vi "PCC Main.vi"(10 "Data Type DVRs":T1, 11 "Config Folder":path) -> ()   [LabVIEW 2018]
uses:
  Controls/State Transition Loop Selector.ctl
  Controls/DDS State.ctl
  <vilib>/ORNL/CSEISMIC DDS/CSEISMIC DDS Base/Data Types/Controls/DeviceID.ctl
  Controls/Data Type DVRs.ctl
  <vilib>/ORNL/CSEISMIC DDS/CSEISMIC DDS Base/Data Types/PCC_Transition.ctl
  <vilib>/ORNL/CSEISMIC DDS/CSEISMIC DDS Base/Data Types/Controls/Timestamp.ctl
  <vilib>/ORNL/CSEISMIC DDS/CSEISMIC DDS Base/Data Types/DER_setGenerationMode.ctl
  <vilib>/ORNL/CSEISMIC DDS/CSEISMIC DDS Base/Data Types/Controls/Generation Mode.ctl
  <vilib>/ORNL/CSEISMIC DDS/CSEISMIC DDS Base/Data Types/IED_Status.ctl
  <vilib>/ORNL/CSEISMIC DDS/CSEISMIC DDS Base/Data Types/DER_VF.ctl
  <vilib>/ORNL/CSEISMIC DDS/CSEISMIC DDS Base/Data Types/SmartRelay_Measurement.ctl
  5fae7271-6999-4ee3-adec-77b7e82a9117.vi
  0c60829f-05e1-488a-9307-f5885f688830.vi
  d2d44614-09ee-478f-a8ad-1eeb43ba122a.vi
  90de438a-d49d-4198-a24f-55d882466989.vi
  1e39ed10-ef24-4d6c-8bee-b3eb3189697a.vi
  ae37c20a-06b2-40c0-9558-581a6213f2f7.vi
  c6f44c25-c2e0-4f56-a5f0-2cf136f07edc.vi
  86f4f49e-388a-4250-a9a8-ce7cd87dfdd2.vi
  05904c7c-c053-4fcf-9d3f-90a477ff682e.vi
  6fac8efd-f310-42bf-8d4e-08964d51a696.vi
  85c23227-e024-4d6f-8611-baa9cc794223.vi
  278e74c7-9ea8-40bf-a49e-ca8128e71b27.vi
  9b8a6be7-b97e-4c02-9044-44fe14d12b33.vi
  Global Variables/Stop (Global).vi
  Global Variables/DDS States (Global).vi
  Global Variables/Manual Control (Global).vi
  Global Variables/Measurements (Global).vi
  <vilib>/ORNL/CSEISMIC DDS/CSEISMIC DDS Base/CSEISMIC DDS.lvclass
  <vilib>/ptbypt/NI_PtbyPt.lvlib
  <vilib>/Analysis/NI_AALBase.lvlib
panel:
  out "Switch Closed?":bool=TRUE
  out "VF DeviceID":T2
  out "MicrogridID":u8
  out "Error in DDS Loop":bool
  out "DDS Error out":errorcluster
  out "DDS State":T3
  out "DDS loop time":u32=100
  out "Error in State Transition Loop":bool
  out "DDS state m/c loop time":u32=100
  out "Trans State":T4
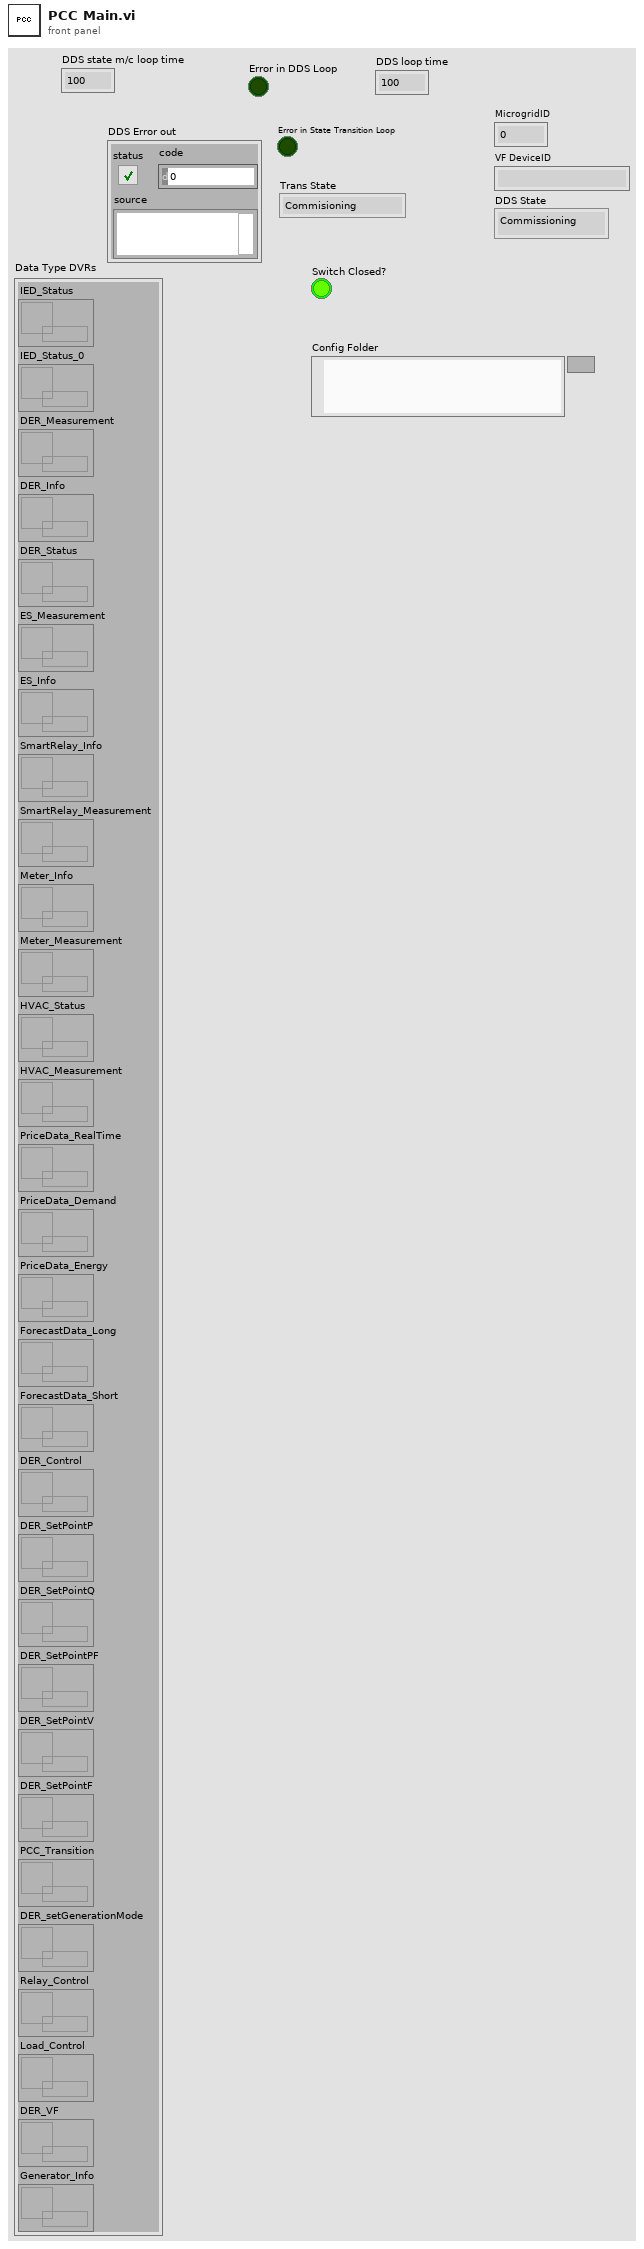
[diagram p1: front panel]
types:
  T1 = typedef "Data Type DVRs.ctl" = cluster{"IED_Status":refnum<data-value>, "IED_Status_0":refnum<data-value>, "DER_Measurement":refnum<data-value>, "DER_Info":refnum<data-value>, "DER_Status":refnum<data-value>, "ES_Measurement":refnum<data-value>, "ES_Info":refnum<data-value>, "SmartRelay_Info":refnum<data-value>, "SmartRelay_Measurement":refnum<data-value>, "Meter_Info":refnum<data-value>, "Meter_Measurement":refnum<data-value>, "HVAC_Status":refnum<data-value>, "HVAC_Measurement":refnum<data-value>, "PriceData_RealTime":refnum<data-value>, "PriceData_Demand":refnum<data-value>, "PriceData_Energy":refnum<data-value>, "ForecastData_Long":refnum<data-value>, "ForecastData_Short":refnum<data-value>, "DER_Control":refnum<data-value>, "DER_SetPointP":refnum<data-value>, "DER_SetPointQ":refnum<data-value>, "DER_SetPointPF":refnum<data-value>, "DER_SetPointV":refnum<data-value>, "DER_SetPointF":refnum<data-value>, "PCC_Transition":refnum<data-value>, "DER_setGenerationMode":refnum<data-value>, "Relay_Control":refnum<data-value>, "Load_Control":refnum<data-value>, "DER_VF":refnum<data-value>, "Generator_Info":refnum<data-value>}
  T2 = typedef "CSEISMIC DDS.lvlib/CSEISMIC DDS.lvclass/DeviceID.ctl" = string
  T3 = typedef "DDS State.ctl" = enum16{"Commissioning", "CheckID", "InitDDS", "ReadDDS", "WriteDDS", "CheckClose", "Close", "Shutdown"}
  T4 = typedef "State Transition Loop Selector.ctl" = enum16{"Commisioning", "Start", "Open", "Closed", "Resynch", "Island", "Close References", "Shutdown"}
  T5 = typedef "Smart Relay Config Settings.ctl" = cluster{"ResynchTimeout":dbl, "IslandTimeout":dbl}
  T6 = typedef "CSEISMIC DDS.lvlib/CSEISMIC DDS.lvclass/SmartRelay_Info.ctl" = cluster{"DeviceID":T2, "LineConfig":u8[], "NominalVoltage(V)":dbl}
  T7 = typedef "CSEISMIC DDS.lvlib/CSEISMIC DDS.lvclass/Timestamp.ctl" = cluster{"Seconds":u64, "Remainder":u64}
  T8 = typedef "CSEISMIC DDS.lvlib/CSEISMIC DDS.lvclass/IED_Status.ctl" = cluster{"DeviceID":T2, "Timestamp":T7, "MicrogridID":u8, "Active":bool, "Inactive":bool, "Error":i32, "Fault":bool, "ErrorString":string}
  T9 = typedef "CSEISMIC DDS.lvlib/CSEISMIC DDS.lvclass/DER_VF.ctl" = cluster{"DeviceID":T2}
  T10 = typedef "CSEISMIC DDS.lvlib/CSEISMIC DDS.lvclass/SmartRelay_Measurement.ctl" = cluster{"DeviceID":T2, "PrimaryVoltage":dbl[], "SecondaryVoltage":dbl[], "Current":dbl[], "RealPower":dbl[], "ReactivePower":dbl[], "LineConfig":u8[], "Frequency":dbl}
  T11 = typedef "CSEISMIC DDS.lvlib/CSEISMIC DDS.lvclass/PCC_Transition.ctl" = cluster{"DeviceID":T2, "Island":bool, "Resynchronize":bool}
  T12 = typedef "CSEISMIC DDS.lvlib/CSEISMIC DDS.lvclass/Generation Mode.ctl" = enum32{"Invalid", "PQ", "Droop", "PV", "PF", "VF"}
  T13 = typedef "CSEISMIC DDS.lvlib/CSEISMIC DDS.lvclass/DER_setGenerationMode.ctl" = cluster{"DeviceID":T2, "Mode":T12}
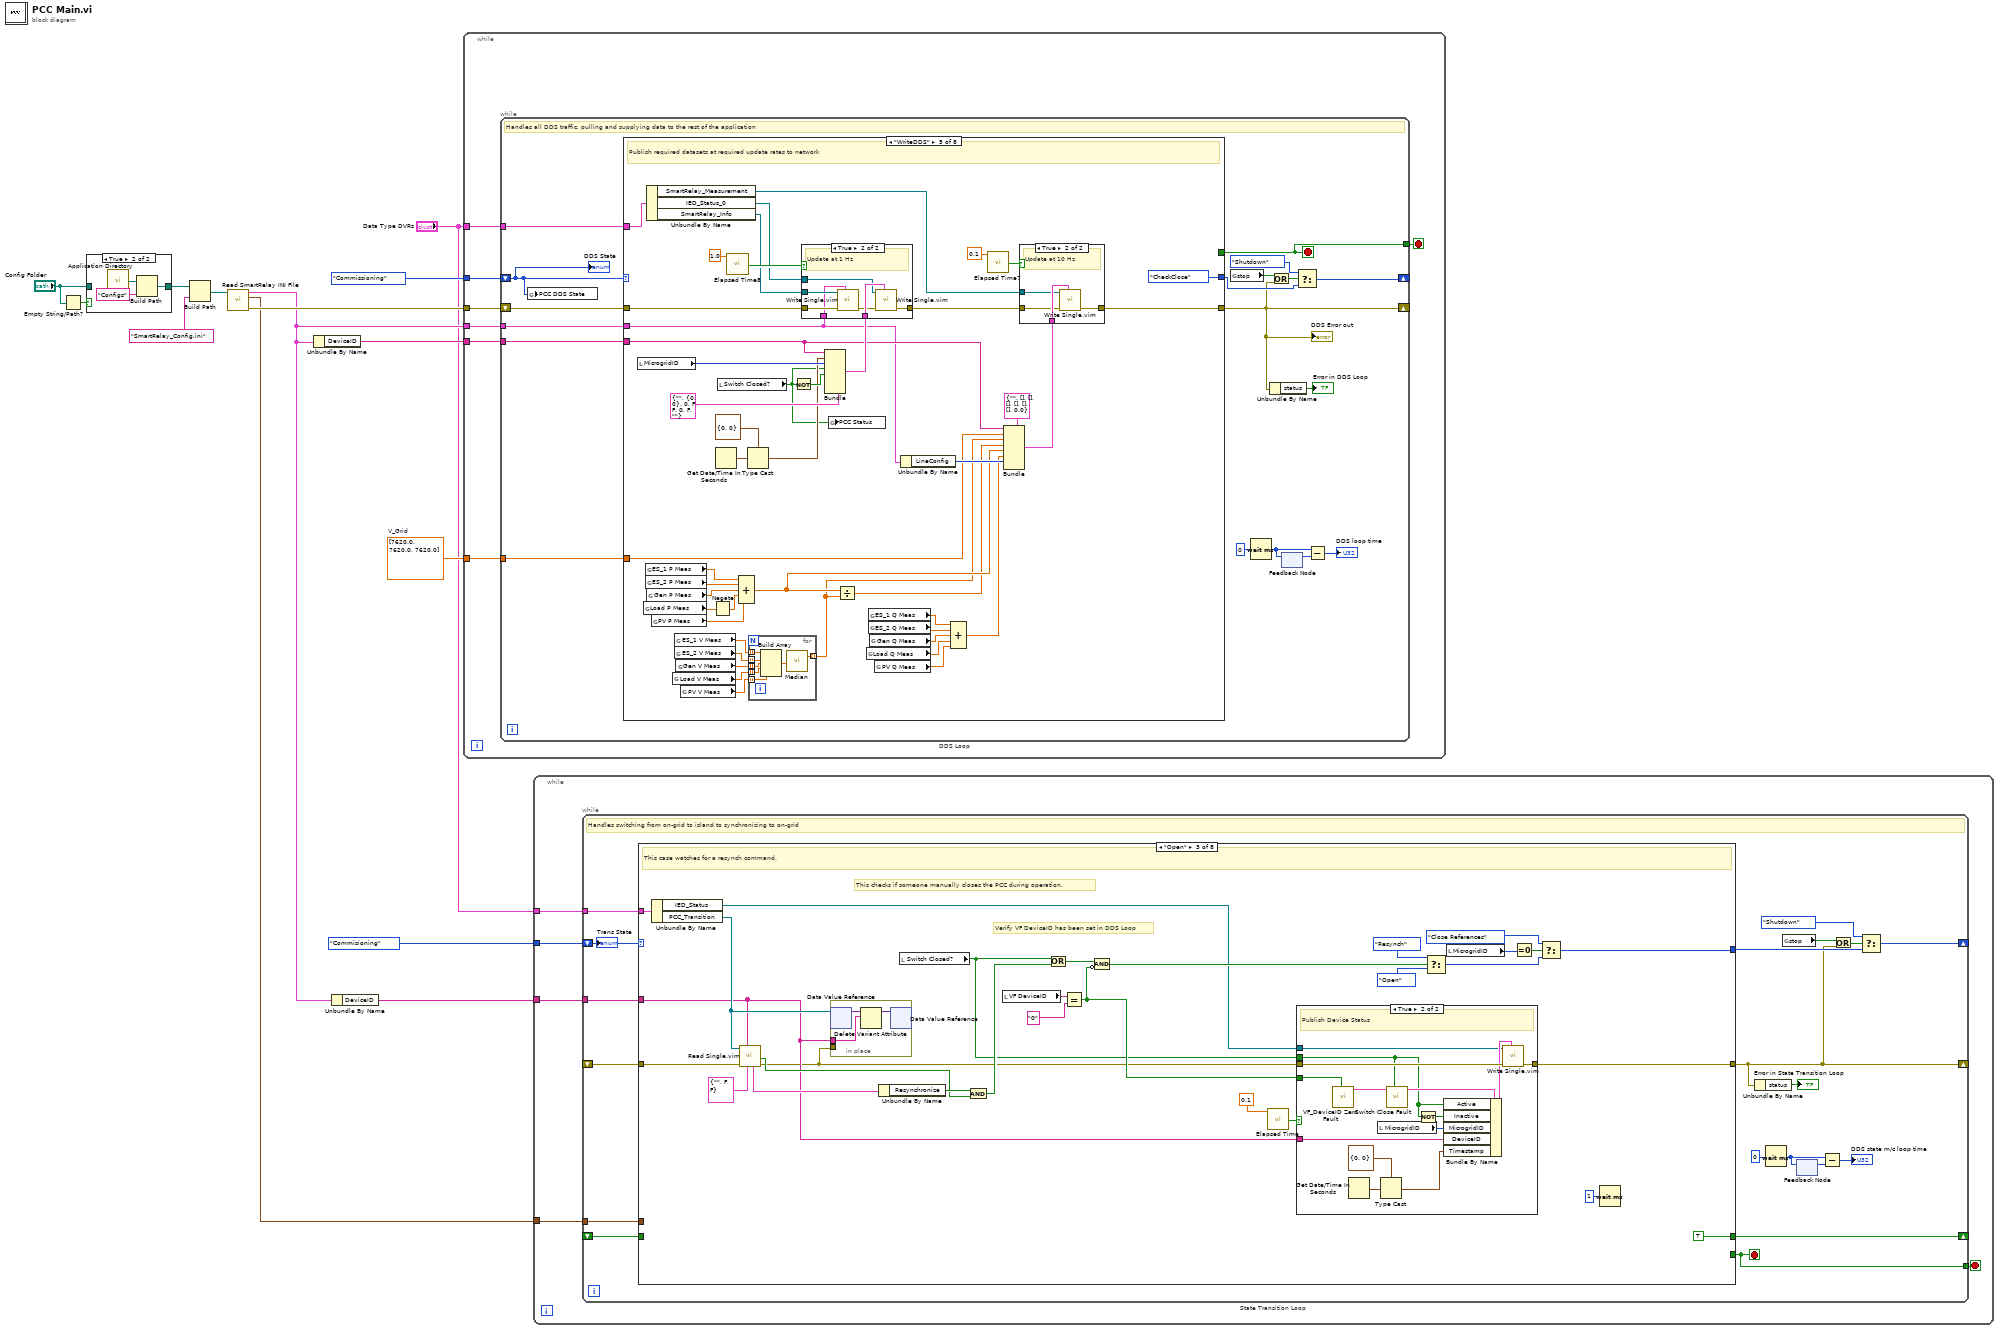
[diagram p0: block diagram]
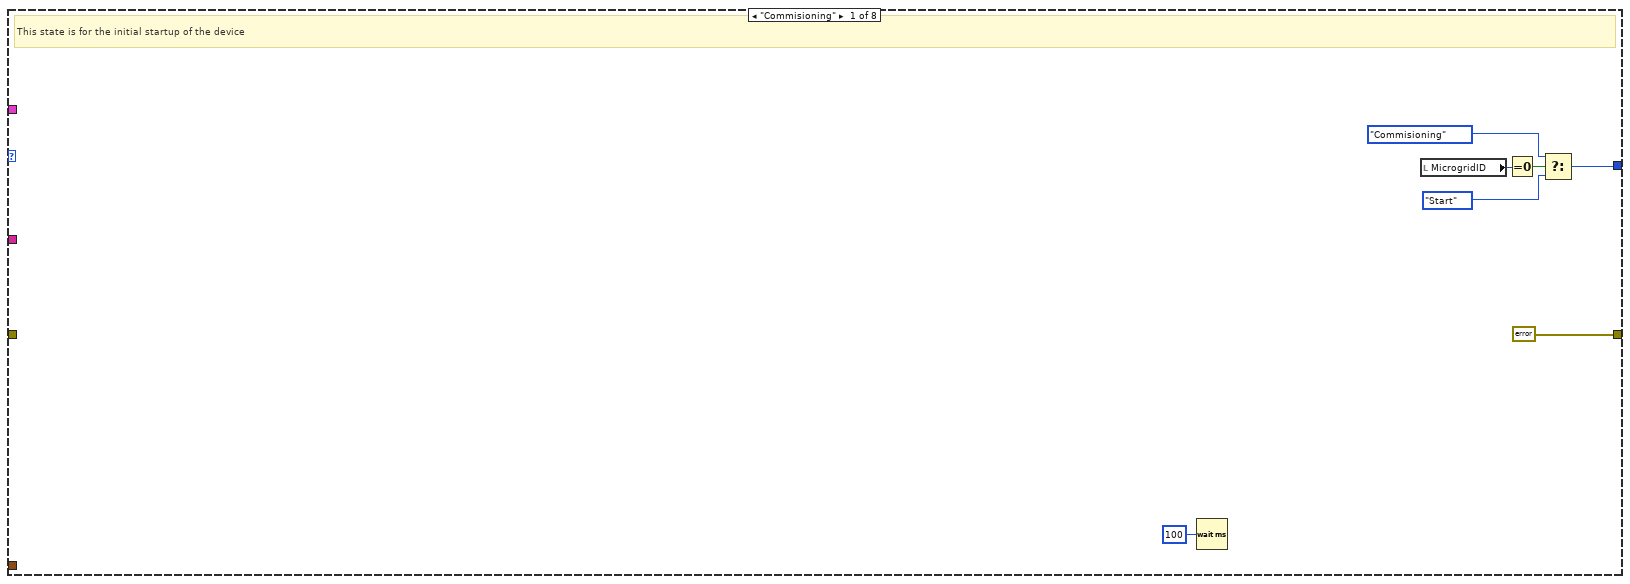
[diagram p2: hidden frame]
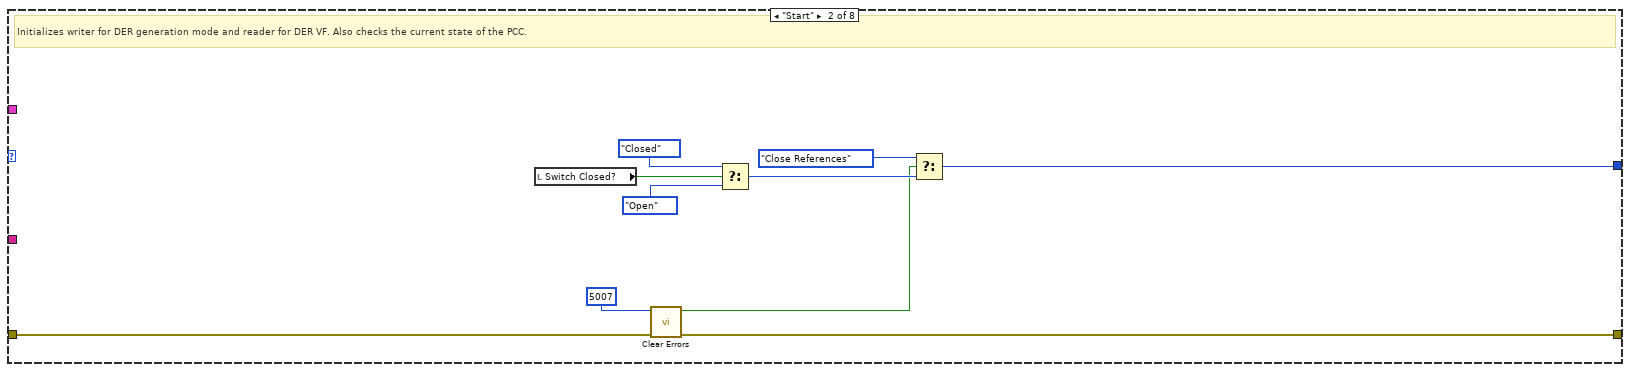
[diagram p3: hidden frame]
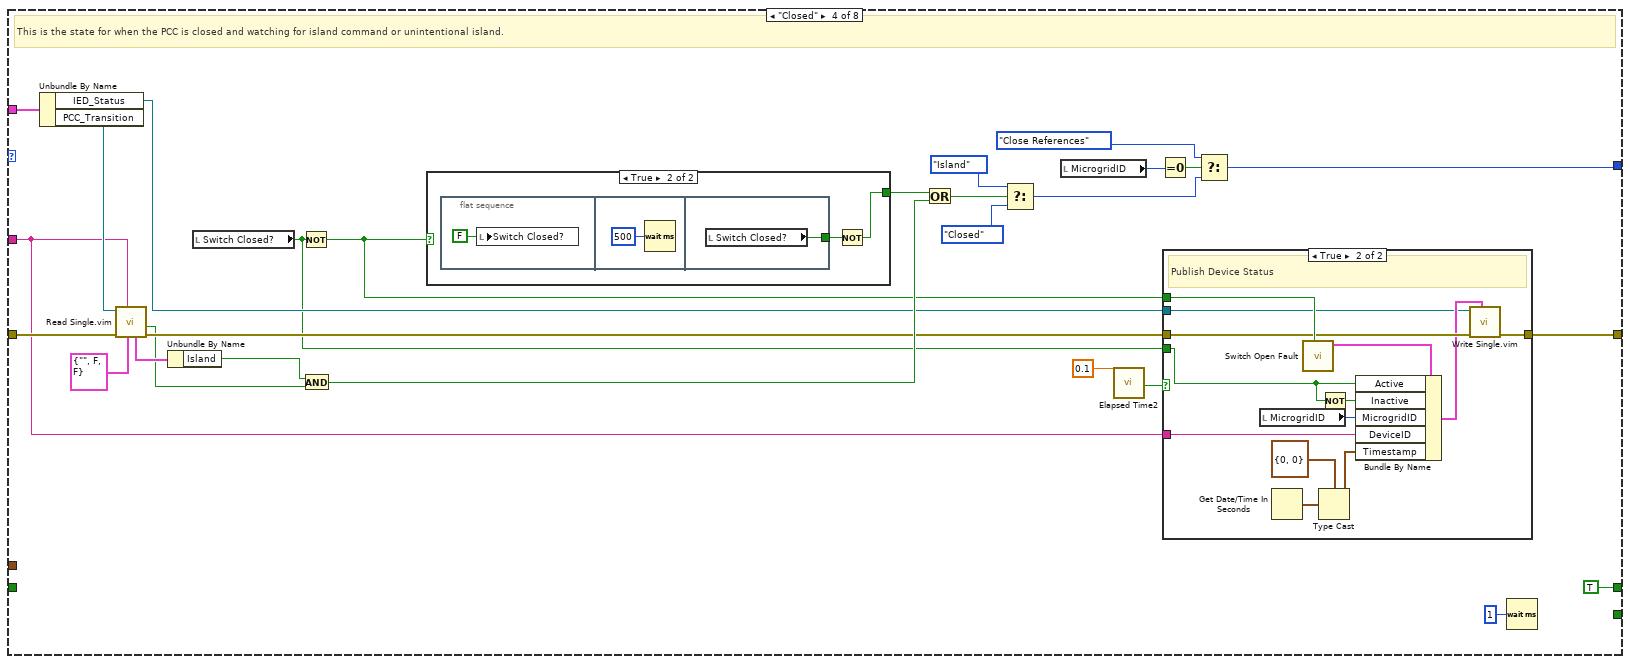
[diagram p5: hidden frame]
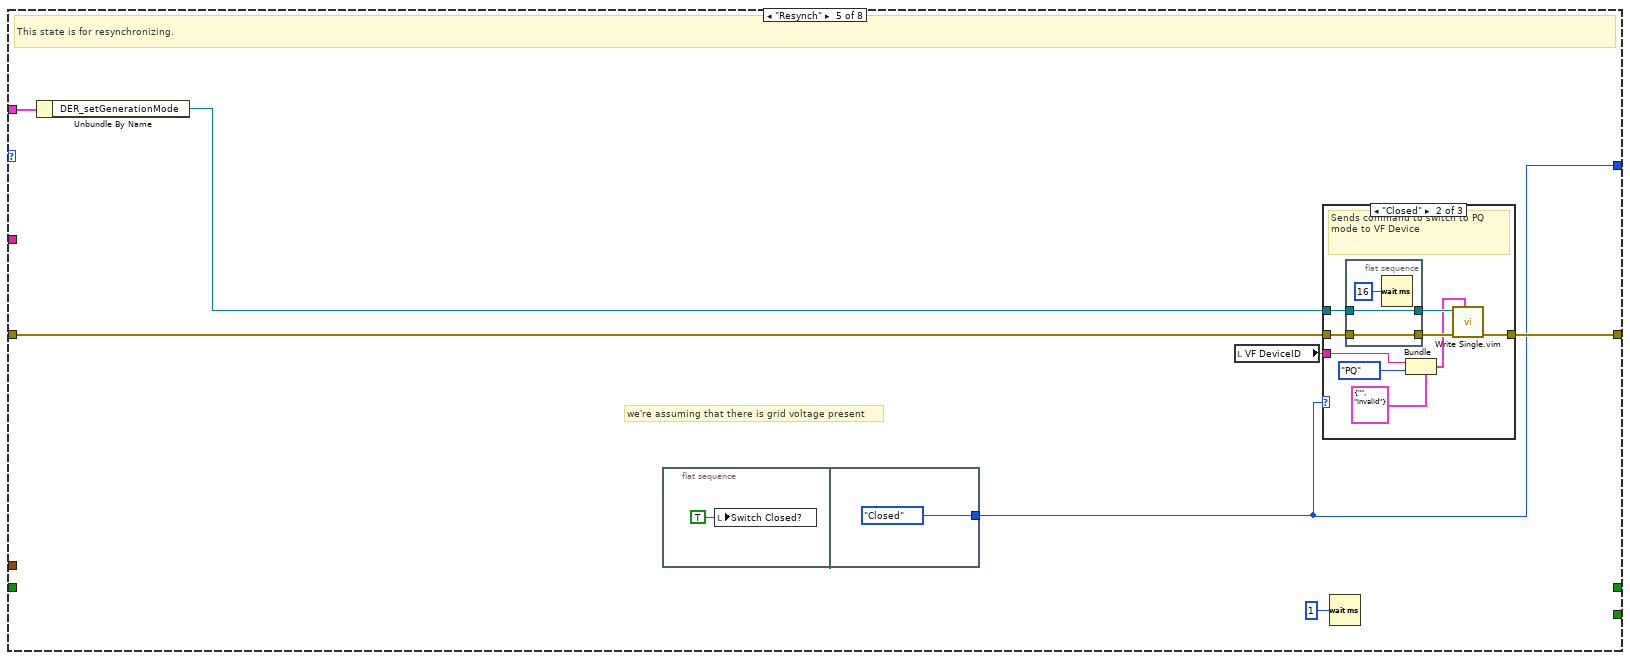
[diagram p8: hidden frame]
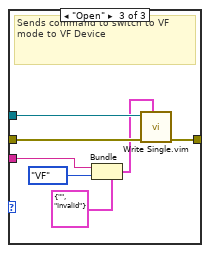
[diagram p10: hidden frame]
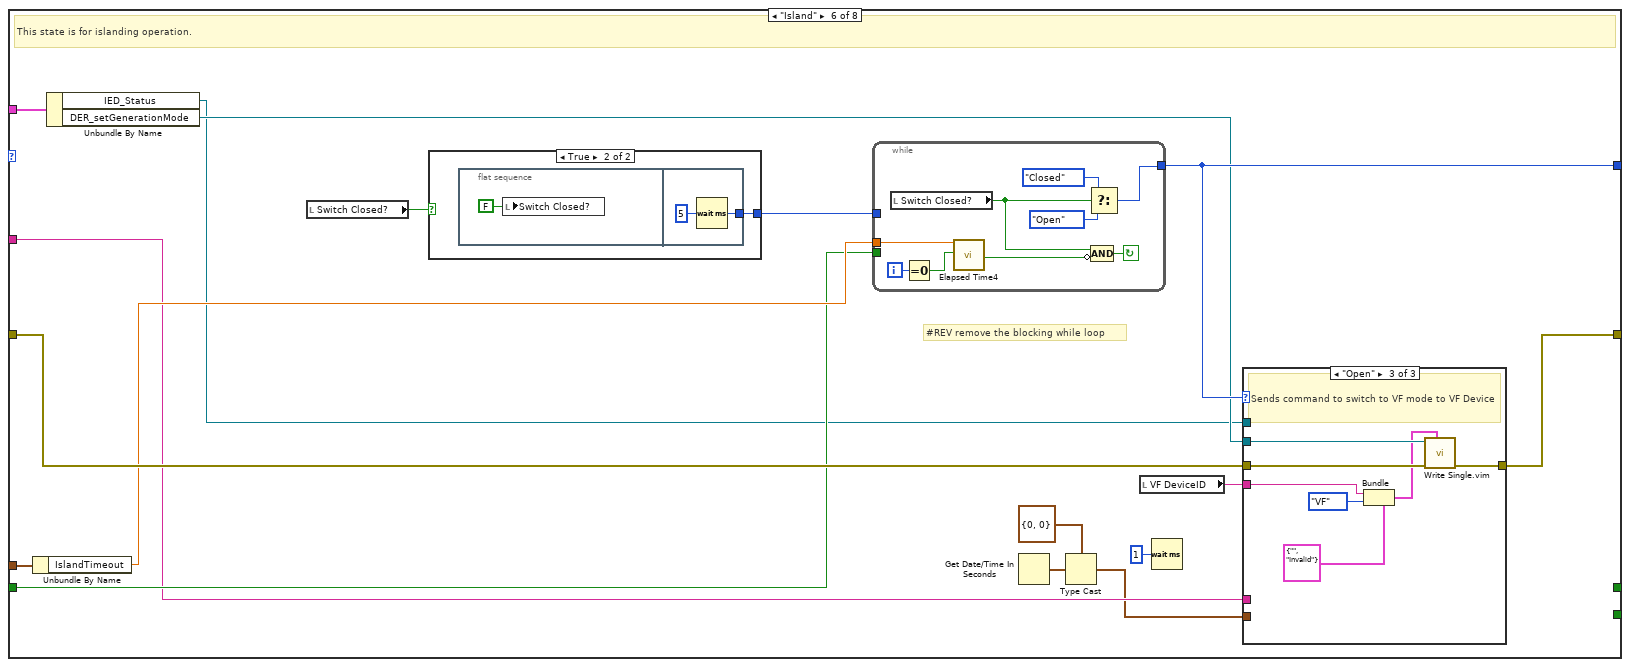
[diagram p11: hidden frame]
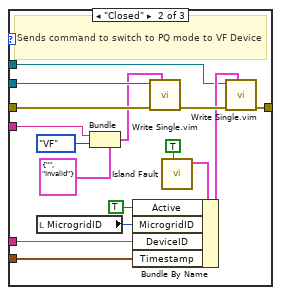
[diagram p13: hidden frame]
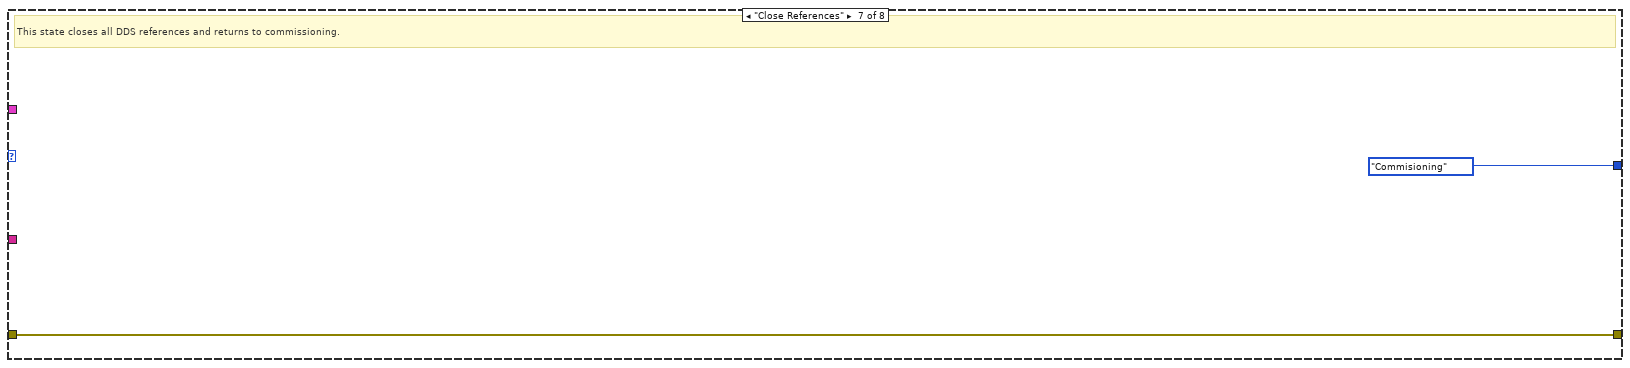
[diagram p15: hidden frame]
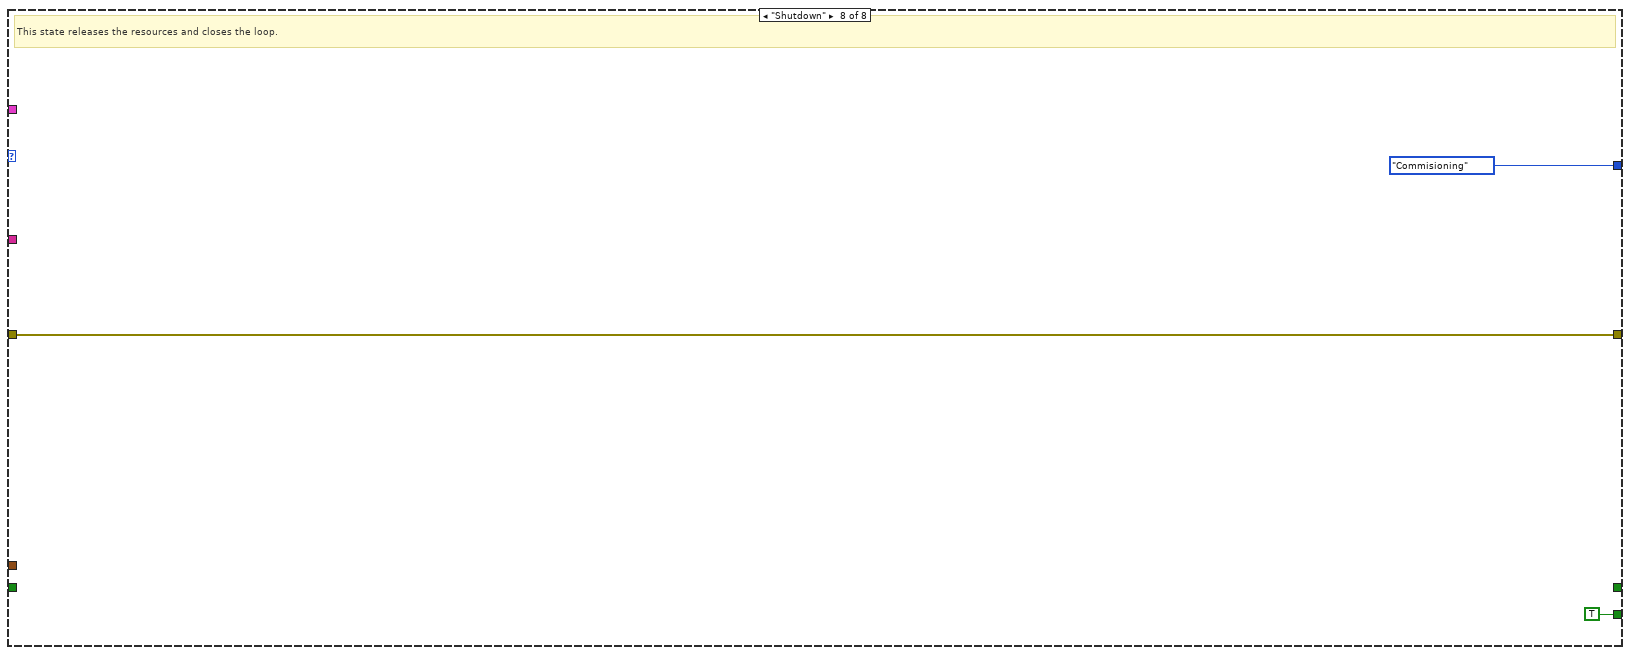
[diagram p16: hidden frame]
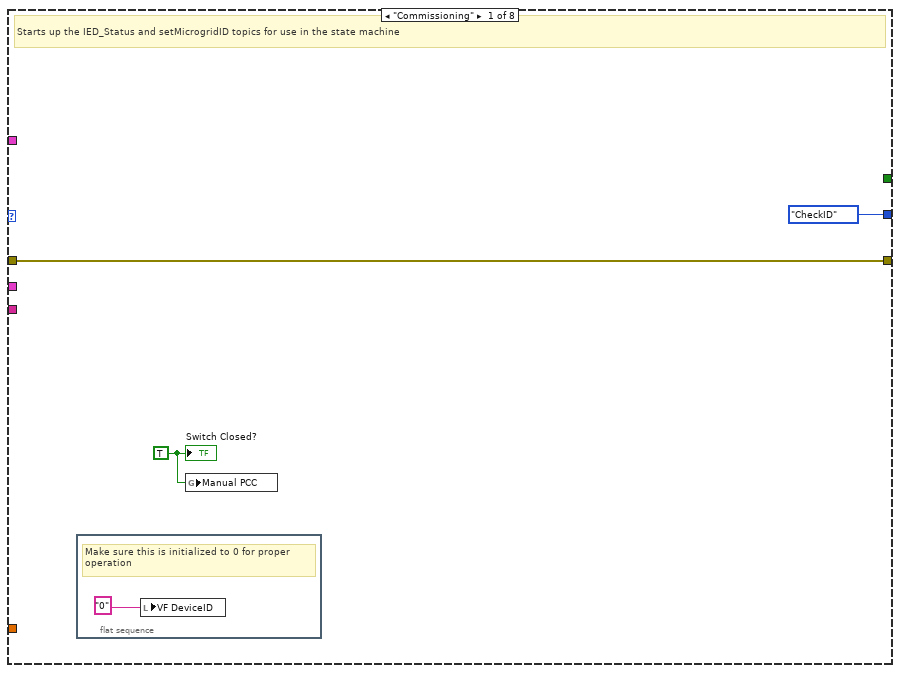
[diagram p17: hidden frame]
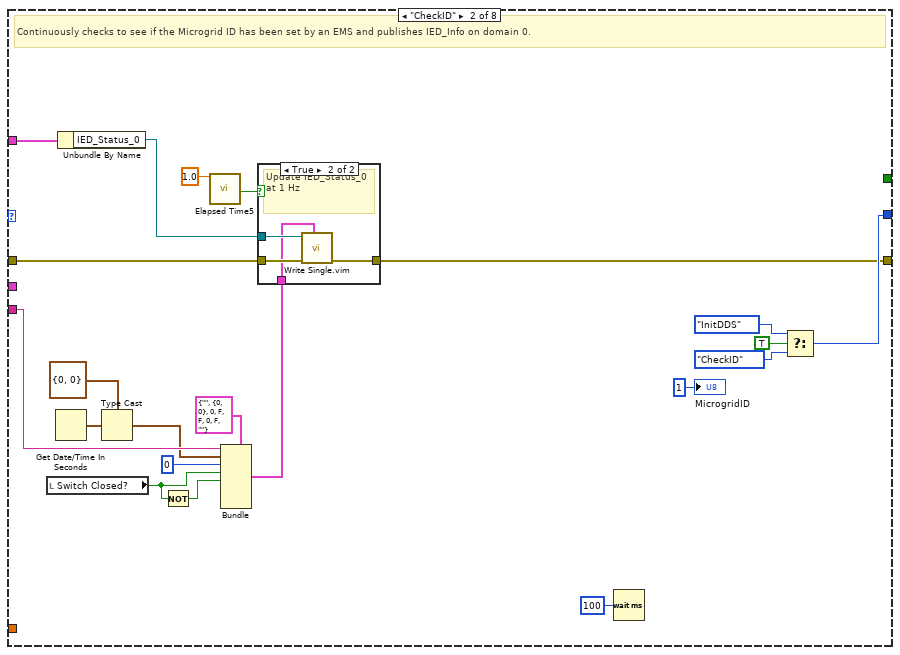
[diagram p18: hidden frame]
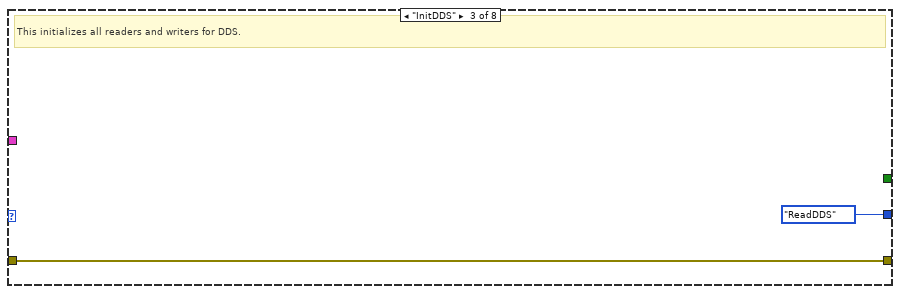
[diagram p20: hidden frame]
diagram:
  w5 = dbl[] [7620.0, 7620.0, 7620.0]  # V_Grid
  n1 = Empty String/Path?(string/path="Config Folder") -> (empty?=w4:bool)
  n2 = case shown="True" w4 {
    tunnel: [w15 w16] -> w2
    tunnel: "Config Folder" -> [w15 _]
    frame False {
    }
    frame True {
      n3 = call <vilib>:"Application Directory.vi"() -> ("Application Directory"=w18:path)
      n4 = Build Path(base path=w18, name or relative path="Configs") -> (appended path=w16:path)
    }
  }
  n5 = Build Path(base path=w2, name or relative path="SmartRelay_Config.ini") -> (appended path=w11:path)
  n6 = call "Read SmartRelay INI File.vi"("Path"=w11) -> ("error out"=w9:errorcluster, "SmartRelay_Config Settings"=w7:T5, "SmartRelay_Info"=w6:T6)  [unwired: 8 in]
  n7 = Unbundle By Name(w6) -> ("DeviceID"=w8:T2)
  n8 = Unbundle By Name(w6) -> ("DeviceID"=w13:T2)
  n9 = while {
    tunnel: w8 -> [w25]
    tunnel: DDS_State."Commissioning" -> [w24]
    tunnel: w9 -> [w23]
    tunnel: w6 -> [w22]
    tunnel: w5 -> [w20]
    tunnel: "Data Type DVRs" -> [w19]
    stop <- w21 stop-if-true
    n10 = while "DDS Loop" {
      shift-right: [w40] -> _
      shift-left: w24 -> [w26]
      tunnel: w25 -> [w43]
      shift-right: [w36] -> _
      shift-left: w23 -> [w42]
      tunnel: w22 -> [w41]
      tunnel: [w34] -> w21
      tunnel: w20 -> [w28]
      tunnel: w19 -> [w29]
      stop <- w34 stop-if-true
      # "Handles all DDS traffic, pulling and supplying data to the rest of the application"
      n11 = global write "DDS States (Global).vi" "PCC DDS State"(w26) -> ()
      n12 = case shown="\"WriteDDS\"" w26 {
        tunnel: [DDS_State."CheckID" w64 DDS_State."ReadDDS" w93 DDS_State."CheckClose" w170 DDS_State."Commissioning" ("f") DDS_State."Commissioning" ("f")] -> w39
        tunnel: w29 -> [_ w50 _ w90 w106 _ _ _]
        tunnel: [w45 w52 w74 w85 w141 w169 w175 w180] -> w36
        tunnel: w43 -> [_ w67 _ _ w142 _ _ _]
        tunnel: w42 -> [w45 w53 w74 w85 w146 w169 w175 w180]
        tunnel: w41 -> [_ _ _ _ w136 _ _ _]
        tunnel: [_ _ _ _ _ _ _ TRUE] -> w34
        tunnel: w28 -> [_ _ _ _ w113 _ _ _]
        frame "Commissioning" {
          w44 = TRUE
          # "Starts up the IED_Status and setMicrogridID topics for use in the state machine"
          n13 = flat-sequence {
            frame #0 {
              # "Make sure this is initialized to 0 for proper operation"
              n14 = local write "VF DeviceID"(T2 "0" ("VF DeviceID")) -> ()
            }
          }
          n15 = global write "Manual Control (Global).vi" "Manual PCC"(w44) -> ()
          "Switch Closed?" <- w44
        }
        frame "CheckID" {
          # "Continuously checks to see if the Microgrid ID has been set by an EMS and publishes IED_Info on domain 0."
          n16 = local read "Switch Closed?"() -> (w56:bool)
          n17 = Get Date/Time In Seconds() -> (seconds since 1Jan1904=w60:timestamp)
          n18 = Unbundle By Name(w50) -> ("IED_Status_0"=w49:refnum<data-value>)
          n19 = Type Cast(type=T7 {"Seconds"=0, "Remainder"=0} ("Timestamp"), x=w60) -> (*(type *) &x=w57:T7)
          n20 = Not(x=w56) -> (.not. x?=w59:bool)
          n21 = call "Elapsed Time5"("Time Target (s)"=1.0) -> ("Time has Elapsed"=w48:bool)  [unwired: 11 in, 7 out]
          n22 = Bundle(cluster=T8 {"DeviceID"="", "Timestamp"={"Seconds"=0, "Remainder"=0}, "MicrogridID"=0, "Active"=FALSE, "Inactive"=FALSE, "Error"=0, "Fault"=FALSE, "ErrorString"=""} ("output cluster"), "DeviceID"=w67, "Timestamp"=w57, "MicrogridID"=u8 0, "Active"=w56, "Inactive"=w59) -> (w51:T8)  [unwired: 3 in]
          n23 = case shown="True" w48 {
            tunnel: w51 -> [_ w70]
            tunnel: [w69 w71] -> w52
            tunnel: w53 -> [w69 w72]
            tunnel: w49 -> [_ w73]
            frame False {
            }
            frame True {
              # "Update IED_Status_0 at 1 Hz"
              n24 = call "Write Single.vim"("Data Element"=w70, "error in"=w72, "Data DVR"=w73) -> ("dup error out"=w71:errorcluster)  [unwired: 8 in]
            }
          }
          n25 = Wait (ms)(milliseconds to wait=u32 100) -> ()  [unwired: 1 out]
          n26 = Select(t=DDS_State."InitDDS", s=TRUE, f=DDS_State."CheckID") -> (s? t:f=w64:T3)
          "MicrogridID" <- u8 1 ("MicrogridID")
        }
        frame "InitDDS" {
          # "This initializes all readers and writers for DDS."
        }
        frame "ReadDDS" {
          # "Read device datasets from network and pass valid values to FPGA layer"
          n27 = Unbundle By Name(w90) -> ("DER_VF"=w84:refnum<data-value>)
          n28 = global read "Manual Control (Global).vi" "Manual PCC"() -> (w76:bool)
          n29 = in-place {
            in-place-border: [w101] -> w88
            # "Get variant from DVR for reading"
            n30 = in-place-dvr #1(w84) -> (w101:variant)  [unwired: 1 out]
            n31 = in-place-dvr #1(w101) -> ()  [unwired: 2 out]
          }
          n32 = First Call?() -> (First Call?: T/F=w79:bool)
          n33 = call <vilib>:"Boolean Crossing PtByPt.vi"("initialize"=w79, "direction"=enum16{"either", "false-true", "true-false"}."either", "input"=w76) -> ("crossing"=w77:bool)
          n34 = case shown="True" w77 {
            tunnel: w76 -> [_ w96]
            frame False {
            }
            frame True {
              n35 = local write "Switch Closed?"(w96) -> ()
            }
          }
          n36 = Get Variant Attribute(Variant=w88) -> (names=w87:string[])  [unwired: 3 in, 3 out]
          n37 = for {
            tunnel: T9 {"DeviceID"=""} ("DER_VF") -> [w100]
            tunnel: w88 -> [w99]
            tunnel: w87 -> [w98] mode=indexing
            tunnel: [w97] -> w86
            n38 = Get Variant Attribute(Variant=w99, name=w98, default value (empty Variant)=w100) -> (value=w97:T9)  [unwired: 1 in, 3 out]
          }
          n39 = Unbundle By Name(w86) -> ("DeviceID"=w82:T2)
          n40 = Empty String/Path?(string/path=w82) -> (empty?=w83:bool)
          n41 = Select(t=T2 "0", s=w83, f=w82) -> (s? t:f=→"VF DeviceID":T2)
          n42 = Wait (ms)(milliseconds to wait=u32 100) -> ()  [unwired: 1 out]
          n43 = Select(t=DDS_State."Close", s=FALSE, f=DDS_State."WriteDDS") -> (s? t:f=w93:T3)
        }
        frame "WriteDDS" {
          # "Publish required datasets at required update rates to network"
          n44 = local read "MicrogridID"() -> (w131:u8)
          n45 = global read "Measurements (Global).vi" "Load P Meas"() -> (w108:dbl[])
          n46 = global read "Measurements (Global).vi" "ES_1 P Meas"() -> (w127:dbl[])
          n47 = global read "Measurements (Global).vi" "ES_2 P Meas"() -> (w126:dbl[])
          n48 = Unbundle By Name(w106) -> ("SmartRelay_Measurement"=w103:refnum<data-value>, "IED_Status_0"=w104:refnum<data-value>, "SmartRelay_Info"=w105:refnum<data-value>)
          n49 = global read "Measurements (Global).vi" "Gen P Meas"() -> (w125:dbl[])
          n50 = global read "Measurements (Global).vi" "PV P Meas"() -> (w124:dbl[])
          n51 = global read "Measurements (Global).vi" "Load V Meas"() -> (w115:dbl[])
          n52 = global read "Measurements (Global).vi" "ES_1 V Meas"() -> (w118:dbl[])
          n53 = global read "Measurements (Global).vi" "ES_2 V Meas"() -> (w117:dbl[])
          n54 = global read "Measurements (Global).vi" "Gen V Meas"() -> (w116:dbl[])
          n55 = global read "Measurements (Global).vi" "PV V Meas"() -> (w114:dbl[])
          n56 = Negate(x=w108) -> (-x=w107:dbl[])
          n57 = Get Date/Time In Seconds() -> (seconds since 1Jan1904=w129:timestamp)
          n58 = local read "Switch Closed?"() -> (w102:bool)
          n59 = call "Elapsed Time8"("Time Target (s)"=1.0) -> ("Time has Elapsed"=w137:bool)  [unwired: 11 in, 7 out]
          n60 = Compound Arithmetic op=ADD(w127, w126, w125, w107, w124) -> (w111:dbl[])
          n61 = Type Cast(type=T7 {"Seconds"=0, "Remainder"=0} ("Timestamp"), x=w129) -> (*(type *) &x=w128:T7)
          n62 = for {
            tunnel: w118 -> [w154] mode=indexing
            tunnel: w117 -> [w153] mode=indexing
            tunnel: w116 -> [w152] mode=indexing
            tunnel: w115 -> [w151] mode=indexing
            tunnel: w114 -> [w150] mode=indexing
            tunnel: [w148] -> w109 mode=indexing
            n63 = Build Array(w154, w153, w152, w151, w150) -> (w149:dbl[])
            n64 = call <vilib>:"Median.vi"("X"=w149) -> ("median"=w148:dbl)  [unwired: 1 out]
          }
          n65 = Not(x=w102) -> (.not. x?=w132:bool)
          n66 = Bundle(cluster=T8 {"DeviceID"="", "Timestamp"={"Seconds"=0, "Remainder"=0}, "MicrogridID"=0, "Active"=FALSE, "Inactive"=FALSE, "Error"=0, "Fault"=FALSE, "ErrorString"=""} ("IED_Status"), "DeviceID"=w142, "Timestamp"=w128, "MicrogridID"=w131, "Active"=w102, "Inactive"=w132) -> (w144:T8)  [unwired: 3 in]
          n67 = case shown="True" w137 {
            tunnel: w146 -> [w160 w167]
            tunnel: [w160 w163] -> w145
            tunnel: w144 -> [_ w165]
            tunnel: w136 -> [_ w161]
            tunnel: w105 -> [_ w166]
            tunnel: w104 -> [_ w164]
            frame False {
            }
            frame True {
              # "Update at 1 Hz"
              n68 = call "Write Single.vim"("Data Element"=w161, "error in"=w167, "Data DVR"=w166) -> ("dup error out"=w162:errorcluster)  [unwired: 8 in]
              n69 = call "Write Single.vim"("Data Element"=w165, "error in"=w162, "Data DVR"=w164) -> ("dup error out"=w163:errorcluster)  [unwired: 8 in]
            }
          }
          n70 = global write "Measurements (Global).vi" "PCC Status"(w102) -> ()
          n71 = Divide(x=w111, y=w109) -> (x/y=w110:dbl[])
          n72 = global read "Measurements (Global).vi" "Load Q Meas"() -> (w120:dbl[])
          n73 = global read "Measurements (Global).vi" "ES_1 Q Meas"() -> (w123:dbl[])
          n74 = global read "Measurements (Global).vi" "ES_2 Q Meas"() -> (w122:dbl[])
          n75 = global read "Measurements (Global).vi" "Gen Q Meas"() -> (w121:dbl[])
          n76 = global read "Measurements (Global).vi" "PV Q Meas"() -> (w119:dbl[])
          n77 = Unbundle By Name(w136) -> ("LineConfig"=w135:u8[])
          n78 = Compound Arithmetic op=ADD(w123, w122, w121, w120, w119) -> (w112:dbl[])
          n79 = call "Elapsed Time7"("Time Target (s)"=0.1) -> ("Time has Elapsed"=w139:bool)  [unwired: 11 in, 7 out]
          n80 = Bundle(cluster=T10 {"DeviceID"="", "PrimaryVoltage"=[], "SecondaryVoltage"=[], "Current"=[], "RealPower"=[], "ReactivePower"=[], "LineConfig"=[], "Frequency"=0.0} ("SmartRelay_Measurement"), "DeviceID"=w142, "PrimaryVoltage"=w113, "SecondaryVoltage"=w109, "Current"=w110, "RealPower"=w111, "ReactivePower"=w112, "LineConfig"=w135) -> (w143:T10)  [unwired: 1 in]
          n81 = case shown="True" w139 {
            tunnel: w145 -> [w155 w158]
            tunnel: w143 -> [_ w159]
            tunnel: [w155 w157] -> w141
            tunnel: w103 -> [_ w156]
            frame False {
            }
            frame True {
              # "Update at 10 Hz"
              n82 = call "Write Single.vim"("Data Element"=w159, "error in"=w158, "Data DVR"=w156) -> ("dup error out"=w157:errorcluster)  [unwired: 8 in]
            }
          }
        }
        frame "CheckClose" {
          # "Check to see if MicrogridID has been reset to 0, releasing the device from Microgrid control"
          n83 = Select(t=DDS_State."Close", s=FALSE, f=DDS_State."ReadDDS") -> (s? t:f=w170:T3)
        }
        frame "Close" {
          # "Set MicrogridID and VF DeviceID to 0 in order for State Transition Loop to function correctly."
          # "Release resources associated with microgrid ID, deactivate device, and return to CheckID state"
          n84 = local write "MicrogridID"(u8 0 ("MicrogridID")) -> ()
          n85 = local write "VF DeviceID"(T2 "0" ("VF DeviceID")) -> ()
        }
        frame "Shutdown" {
          # "Set MicrogridID and VF DeviceID to 0 in order for State Transition Loop to function correctly."
          # "Release resources and stop loop"
          n86 = local write "MicrogridID"(u8 0 ("MicrogridID")) -> ()
          n87 = local write "VF DeviceID"(T2 "0" ("VF DeviceID")) -> ()
        }
      }
      "DDS Error out" <- w36
      n88 = global read "Stop (Global).vi" "stop"() -> (w27:bool)
      n89 = Wait (ms)(milliseconds to wait=u32 0) -> (millisecond timer value=w32:u32)
      n90 = Unbundle By Name(w36) -> ("status"=→"Error in DDS Loop":bool)
      n91 = Or(x=w27, y=w36) -> (x .or. y?=w37:bool)
      n92 = feedback #2() -> (w31:u32)  [unwired: 1 in]
      n93 = feedback-in #2(w32) -> ()
      n94 = Select(t=DDS_State."Shutdown", s=w37, f=w39) -> (s? t:f=w40:T3)
      n95 = Subtract(x=w32, y=w31) -> (x-y=→"DDS loop time":u32)
      "DDS State" <- w26
    }
  }
  n96 = while {
    tunnel: State_Transition_Loop_Selector."Commisioning" -> [w186]
    tunnel: w7 -> [w185]
    tunnel: "Data Type DVRs" -> [w183]
    tunnel: w13 -> [w182]
    stop <- w184 stop-if-true
    n97 = while "State Transition Loop" {
      shift-right: [w200] -> _
      shift-left: w186 -> [w205]
      shift-right: [w198] -> _
      shift-left: _ -> [w204]
      shift-right: [w196] -> _
      shift-left: _ -> [w197]
      tunnel: w185 -> [w195]
      tunnel: [w194] -> w184
      tunnel: w182 -> [w188]
      tunnel: w183 -> [w189]
      stop <- w194 stop-if-true
      # "Handles switching from on-grid to island to synchronizing to on-grid"
      n98 = case shown="\"Open\"" w205 {
        tunnel: [errorcluster {"status"=FALSE, "code"=0, "source"=""} ("error out") w219 w237 w283 w321 w359 w401 w402] -> w198
        tunnel: w204 -> [_ w220 w231 w276 w322 w361 w401 w402]
        tunnel: [w209 w216 w251 w296 w319 w360 State_Transition_Loop_Selector."Commisioning" State_Transition_Loop_Selector."Commisioning"] -> w199
        tunnel: [_ _ _ _ _ _ _ TRUE] -> w194
        tunnel: w197 -> [_ _ _ _ _ w356 _ _]
        tunnel: [_ _ TRUE TRUE _ _ _ _] -> w196
        tunnel: w195 -> [_ _ _ _ _ w358 _ _]
        tunnel: w189 -> [_ _ w230 w277 w318 w351 _ _]
        tunnel: w188 -> [_ _ w224 w272 _ w352 _ _]
        frame "Commisioning" {
          # "This state is for the initial startup of the device"
          n99 = Wait (ms)(milliseconds to wait=u32 100) -> ()  [unwired: 1 out]
          n100 = local read "MicrogridID"() -> (w207:u8)
          n101 = Equal To 0?(x=w207) -> (x = 0?=w206:bool)
          n102 = Select(t=State_Transition_Loop_Selector."Commisioning", s=w206, f=State_Transition_Loop_Selector."Start") -> (s? t:f=w209:T4)
        }
        frame "Start" {
          # "Initializes writer for DER generation mode and reader for DER VF. Also checks the current state of the PCC."
          n103 = local read "Switch Closed?"() -> (w213:bool)
          n104 = call <vilib>:"Clear Errors.vi"("error in (no error)"=w220, "specific error code to clear (0: all)"=5007) -> ("error out"=w219:errorcluster, "specific error cleared?"=w214:bool)  [unwired: 4 in]
          n105 = Select(t=State_Transition_Loop_Selector."Closed", s=w213, f=State_Transition_Loop_Selector."Open") -> (s? t:f=w218:T4)
          n106 = Select(t=State_Transition_Loop_Selector."Close References", s=w214, f=w218) -> (s? t:f=w216:T4)
        }
        frame "Open" {
          # "Verify VF DeviceID has been set in DDS Loop"
          # "This checks if someone manually closes the PCC during operation."
          # "This case watches for a resynch command."
          n107 = Unbundle By Name(w230) -> ("IED_Status"=w226:refnum<data-value>, "PCC_Transition"=w225:refnum<data-value>)
          n108 = call "Read Single.vim"("Data Type"=T11 {"DeviceID"="", "Island"=FALSE, "Resynchronize"=FALSE} ("PCC_Transition"), "DeviceID"=w224, "error in"=w231, "Data DVR"=w225) -> ("dup error out"=w223:errorcluster, "Valid"=w227:bool, "Data Element"=w228:T11)  [unwired: 5 in]
          n109 = in-place {
            in-place-border: w224 -> [w252]
            in-place-border: w223 -> [_]
            n110 = in-place-dvr #3(w225) -> (w254:variant)  [unwired: 1 out]
            n111 = Delete Variant Attribute(6:w252, 7:w254) -> (3:w253:variant)  [unwired: 1 in, 2 out]
            n112 = in-place-dvr #3(w253) -> ()  [unwired: 2 out]
          }
          n113 = Unbundle By Name(w228) -> ("Resynchronize"=w246:bool)
          n114 = local read "Switch Closed?"() -> (w232:bool)
          n115 = And(x=w246, y=w227) -> (x .and. y?=w245:bool)
          n116 = local read "VF DeviceID"() -> (w234:T2)
          n117 = Or(x=w232, y=w245) -> (x .or. y?=w241:bool)
          n118 = Equal?(x=w234, y="0") -> (x = y?=w235:bool)
          n119 = Compound Arithmetic op=AND(w241, invert w235) -> (w239:bool)
          n120 = call "Elapsed Time"("Time Target (s)"=0.1) -> ("Time has Elapsed"=w236:bool)  [unwired: 11 in, 7 out]
          n121 = case shown="True" w236 {
            tunnel: w223 -> [w255 w264]
            tunnel: [w255 w263] -> w237
            tunnel: w224 -> [_ w265]
            tunnel: w235 -> [_ w268]
            tunnel: w232 -> [_ w257]
            tunnel: w226 -> [_ w261]
            frame False {
            }
            frame True {
              # "Publish Device Status"
              n122 = call "VF_DeviceID Zero Fault.vi"("VF DeviceID 0?"=w268) -> ("IED_Status_ID out"=w267:T8)  [unwired: 10 in]
              n123 = Get Date/Time In Seconds() -> (seconds since 1Jan1904=w259:timestamp)
              n124 = local read "MicrogridID"() -> (w269:u8)
              n125 = Type Cast(type=T7 {"Seconds"=0, "Remainder"=0} ("Timestamp"), x=w259) -> (*(type *) &x=w258:T7)
              n126 = call "Switch Close Fault.vi"("Switch Closed?"=w257, "IED_Status_ID in"=w267) -> ("IED_Status_ID out"=w266:T8)  [unwired: 9 in]
              n127 = Not(x=w257) -> (.not. x?=w256:bool)
              n128 = Bundle By Name(cluster=w266, "Active"=w257, "Inactive"=w256, "MicrogridID"=w269, "DeviceID"=w265, "Timestamp"=w258) -> (w262:T8)
              n129 = call "Write Single.vim"("Data Element"=w262, "error in"=w264, "Data DVR"=w261) -> ("dup error out"=w263:errorcluster)  [unwired: 8 in]
            }
          }
          n130 = Select(t=State_Transition_Loop_Selector."Resynch", s=w239, f=State_Transition_Loop_Selector."Open") -> (s? t:f=w247:T4)
          n131 = local read "MicrogridID"() -> (w250:u8)
          n132 = Equal To 0?(x=w250) -> (x = 0?=w249:bool)
          n133 = Select(t=State_Transition_Loop_Selector."Close References", s=w249, f=w247) -> (s? t:f=w251:T4)
          n134 = Wait (ms)(milliseconds to wait=u32 1) -> ()  [unwired: 1 out]
        }
        frame "Closed" {
          # "This is the state for when the PCC is closed and watching for island command or unintentional island."
          n135 = Unbundle By Name(w277) -> ("IED_Status"=w271:refnum<data-value>, "PCC_Transition"=w279:refnum<data-value>)
          n136 = call "Read Single.vim"("Data Type"=T11 {"DeviceID"="", "Island"=FALSE, "Resynchronize"=FALSE} ("PCC_Transition"), "DeviceID"=w272, "error in"=w276, "Data DVR"=w279) -> ("dup error out"=w275:errorcluster, "Valid"=w273:bool, "Data Element"=w274:T11)  [unwired: 5 in]
          n137 = Unbundle By Name(w274) -> ("Island"=w291:bool)
          n138 = local read "Switch Closed?"() -> (w270:bool)
          n139 = Not(x=w270) -> (.not. x?=w281:bool)
          n140 = And(x=w291, y=w273) -> (x .and. y?=w290:bool)
          n141 = case shown="True" w281 {
            selector: w281 -> [w297 _]
            tunnel: [w297 w299] -> w280
            frame False {
            }
            frame True {
              n142 = flat-sequence {
                tunnel: [w302] -> w298
                frame #0 {
                  n143 = local write "Switch Closed?"(FALSE ("Switch Closed?")) -> ()
                }
                frame #1 {
                  n144 = Wait (ms)(milliseconds to wait=u32 500) -> ()  [unwired: 1 out]
                }
                frame #2 {
                  n145 = local read "Switch Closed?"() -> (w302:bool)
                }
              }
              n146 = Not(x=w298) -> (.not. x?=w299:bool)
            }
          }
          n147 = Or(x=w280, y=w290) -> (x .or. y?=w286:bool)
          n148 = Select(t=State_Transition_Loop_Selector."Island", s=w286, f=State_Transition_Loop_Selector."Closed") -> (s? t:f=w292:T4)
          n149 = local read "MicrogridID"() -> (w295:u8)
          n150 = call "Elapsed Time2"("Time Target (s)"=0.1) -> ("Time has Elapsed"=w284:bool)  [unwired: 11 in, 7 out]
          n151 = Equal To 0?(x=w295) -> (x = 0?=w294:bool)
          n152 = case shown="True" w284 {
            tunnel: w275 -> [w303 w312]
            tunnel: [w303 w311] -> w283
            tunnel: w272 -> [_ w313]
            tunnel: w281 -> [_ w315]
            tunnel: w271 -> [_ w309]
            tunnel: w270 -> [_ w304]
            frame False {
            }
            frame True {
              # "Publish Device Status"
              n153 = local read "MicrogridID"() -> (w316:u8)
              n154 = Get Date/Time In Seconds() -> (seconds since 1Jan1904=w307:timestamp)
              n155 = call "Switch Open Fault.vi"("Switch Open?"=w315) -> ("IED_Status_ID out"=w314:T8)  [unwired: 10 in]
              n156 = Type Cast(type=T7 {"Seconds"=0, "Remainder"=0} ("Timestamp"), x=w307) -> (*(type *) &x=w306:T7)
              n157 = Not(x=w304) -> (.not. x?=w305:bool)
              n158 = Bundle By Name(cluster=w314, "Active"=w304, "Inactive"=w305, "MicrogridID"=w316, "DeviceID"=w313, "Timestamp"=w306) -> (w310:T8)
              n159 = call "Write Single.vim"("Data Element"=w310, "error in"=w312, "Data DVR"=w309) -> ("dup error out"=w311:errorcluster)  [unwired: 8 in]
            }
          }
          n160 = Select(t=State_Transition_Loop_Selector."Close References", s=w294, f=w292) -> (s? t:f=w296:T4)
          n161 = Wait (ms)(milliseconds to wait=u32 1) -> ()  [unwired: 1 out]
        }
        frame "Resynch" {
          # "we're assuming that there is grid voltage present"
          # "This state is for resynchronizing."
          n162 = Unbundle By Name(w318) -> ("DER_setGenerationMode"=w317:refnum<data-value>)
          n163 = flat-sequence {
            tunnel: [State_Transition_Loop_Selector."Closed"] -> w319
            frame #0 {
              n164 = local write "Switch Closed?"(TRUE ("Switch Closed?")) -> ()
            }
            frame #1 {
            }
          }
          n165 = local read "VF DeviceID"() -> (w320:T2)
          n166 = case shown="\"Closed\"" w319 {
            tunnel: w317 -> [_ w332 w343]
            tunnel: w322 -> [w326 w334 w341]
            tunnel: w320 -> [_ w335 w344]
            tunnel: [w326 w329 w342] -> w321
            frame "Resynch", Default {
            }
            frame "Closed" {
              # "Sends command to switch to PQ mode to VF Device"
              n167 = flat-sequence {
                tunnel: w334 -> [w338]
                tunnel: [w338] -> w330
                tunnel: w332 -> [w336]
                tunnel: [w336] -> w331
                frame #0 {
                  n168 = Wait (ms)(milliseconds to wait=u32 16) -> ()  [unwired: 1 out]
                }
              }
              n169 = Bundle(cluster=T13 {"DeviceID"="", "Mode"=enum."Invalid"} ("DER_setGenerationMode"), "DeviceID"=w335, "Mode"=Generation_Mode."PQ") -> (w328:T13)
              n170 = call "Write Single.vim"("Data Element"=w328, "error in"=w330, "Data DVR"=w331) -> ("dup error out"=w329:errorcluster)  [unwired: 8 in]
            }
            frame "Open" {
              # "Sends command to switch to VF mode to VF Device"
              n171 = Bundle(cluster=T13 {"DeviceID"="", "Mode"=enum."Invalid"} ("DER_setGenerationMode"), "DeviceID"=w344, "Mode"=Generation_Mode."VF") -> (w340:T13)
              n172 = call "Write Single.vim"("Data Element"=w340, "error in"=w341, "Data DVR"=w343) -> ("dup error out"=w342:errorcluster)  [unwired: 8 in]
            }
          }
          n173 = Wait (ms)(milliseconds to wait=u32 1) -> ()  [unwired: 1 out]
        }
        frame "Island" {
          # "#REV remove the blocking while loop"
          # "This state is for islanding operation."
          n174 = Unbundle By Name(w358) -> ("IslandTimeout"=w357:dbl)
          n175 = Unbundle By Name(w351) -> ("IED_Status"=w349:refnum<data-value>, "DER_setGenerationMode"=w350:refnum<data-value>)
          n176 = local read "Switch Closed?"() -> (w354:bool)
          n177 = case shown="True" w354 {
            tunnel: [_ w396] -> w353
            frame False {
            }
            frame True {
              n178 = flat-sequence {
                tunnel: [w398] -> w396
                frame #0 {
                  n179 = local write "Switch Closed?"(FALSE ("Switch Closed?")) -> ()
                }
                frame #1 {
                  n180 = Wait (ms)(milliseconds to wait=u32 5) -> (millisecond timer value=w398:u32)
                }
              }
            }
          }
          n181 = while {
            tunnel: [w390] -> w360
            tunnel: w357 -> [w395]
            tunnel: w356 -> [_]
            tunnel: w353 -> [_]
            i -> [w389]
            stop <- w394 continue-if-true
            n182 = local read "Switch Closed?"() -> (w387:bool)
            n183 = Equal To 0?(x=w389) -> (x = 0?=w388:bool)
            n184 = call "Elapsed Time4"("Time Target (s)"=w395, "Reset"=w388) -> ("Time has Elapsed"=w393:bool)  [unwired: 10 in, 7 out]
            n185 = Select(t=State_Transition_Loop_Selector."Closed", s=w387, f=State_Transition_Loop_Selector."Open") -> (s? t:f=w390:T4)
            n186 = Compound Arithmetic op=AND(w387, invert w393) -> (w394:bool)
          }
          n187 = Get Date/Time In Seconds() -> (seconds since 1Jan1904=w347:timestamp)
          n188 = Type Cast(type=T7 {"Seconds"=0, "Remainder"=0} ("Timestamp"), x=w347) -> (*(type *) &x=w346:T7)
          n189 = local read "VF DeviceID"() -> (w362:T2)
          n190 = Wait (ms)(milliseconds to wait=u32 1) -> ()  [unwired: 1 out]
          n191 = case shown="\"Open\"" w360 {
            tunnel: w350 -> [_ w372 w382]
            tunnel: w361 -> [w363 w371 w384]
            tunnel: w362 -> [_ w379 w386]
            tunnel: [w363 w368 w383] -> w359
            tunnel: w352 -> [_ w374 _]
            tunnel: w349 -> [_ w366 _]
            tunnel: w346 -> [_ w364 _]
            frame "Resynch", Default {
            }
            frame "Closed" {
              # "Sends command to switch to PQ mode to VF Device"
              n192 = local read "MicrogridID"() -> (w378:u8)
              n193 = Bundle(cluster=T13 {"DeviceID"="", "Mode"=enum."Invalid"} ("DER_setGenerationMode"), "DeviceID"=w379, "Mode"=Generation_Mode."VF") -> (w370:T13)
              n194 = call "Write Single.vim"("Data Element"=w370, "error in"=w371, "Data DVR"=w372) -> ("dup error out"=w369:errorcluster)  [unwired: 8 in]
              n195 = call "Island Fault.vi"("Switch Closed?"=TRUE) -> ("IED_Status_ID out"=w375:T8)  [unwired: 10 in]
              n196 = Bundle By Name(cluster=w375, "Active"=TRUE ("Inactive"), "MicrogridID"=w378, "DeviceID"=w374, "Timestamp"=w364) -> (w367:T8)
              n197 = call "Write Single.vim"("Data Element"=w367, "error in"=w369, "Data DVR"=w366) -> ("dup error out"=w368:errorcluster)  [unwired: 8 in]
            }
            frame "Open" {
              # "Sends command to switch to VF mode to VF Device"
              n198 = Bundle(cluster=T13 {"DeviceID"="", "Mode"=enum."Invalid"} ("DER_setGenerationMode"), "DeviceID"=w386, "Mode"=Generation_Mode."VF") -> (w381:T13)
              n199 = call "Write Single.vim"("Data Element"=w381, "error in"=w384, "Data DVR"=w382) -> ("dup error out"=w383:errorcluster)  [unwired: 8 in]
            }
          }
        }
        frame "Close References" {
          # "This state closes all DDS references and returns to commissioning."
        }
        frame "Shutdown" {
          # "This state releases the resources and closes the loop."
        }
      }
      n200 = Unbundle By Name(w198) -> ("status"=→"Error in State Transition Loop":bool)
      n201 = Wait (ms)(milliseconds to wait=u32 0) -> (millisecond timer value=w192:u32)
      n202 = global read "Stop (Global).vi" "stop"() -> (w187:bool)
      n203 = feedback #4() -> (w191:u32)  [unwired: 1 in]
      n204 = feedback-in #4(w192) -> ()
      n205 = Subtract(x=w192, y=w191) -> (x-y=→"DDS state m/c loop time":u32)
      n206 = Or(x=w187, y=w198) -> (x .or. y?=w202:bool)
      n207 = Select(t=State_Transition_Loop_Selector."Shutdown", s=w202, f=w199) -> (s? t:f=w200:T4)
      "Trans State" <- w205
    }
  }
